vi "多参校准第二步.vi"(11 "校准模式":enum32{"单点校准", "多点校准"}(radio)) -> (1 "标样2浓度输出":dbl, 2 "标样1浓度输出":dbl, 3 "继续执行":bool)   [LabVIEW 2016, in "斯坦道仪器.lvlib"]
panel:
  in  "标样浓度 2":dbl
  in  "标样浓度":dbl
  in  "取消":bool
  in  "下一步":bool
  # "请输入标样一浓度："
  # "请输入标样二浓度："
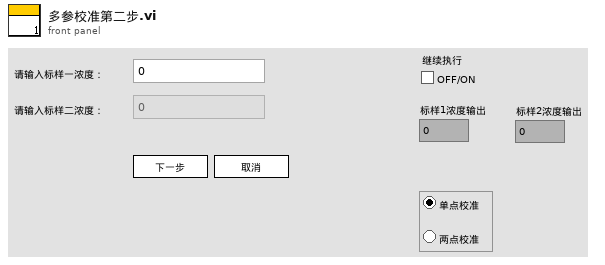
[diagram p1: front panel]
types:
  T1 = enum8{"Enabled", "Disabled", "Disabled and Grayed Out"}
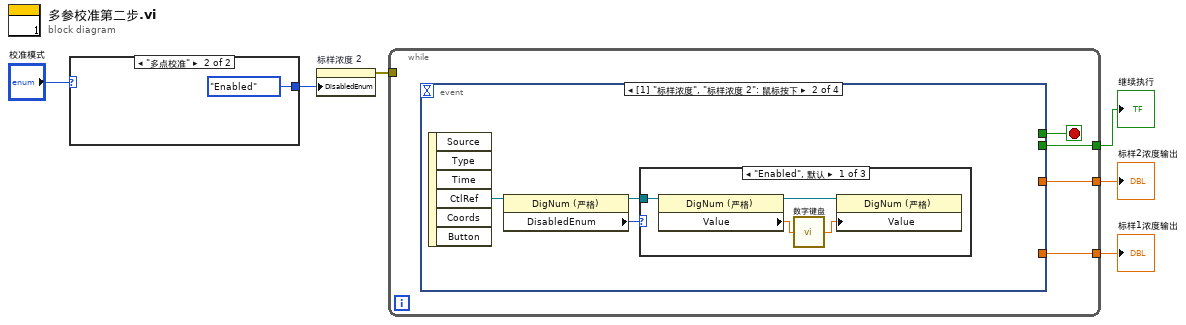
[diagram p0: block diagram]
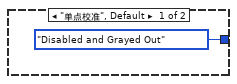
[diagram p2: hidden frame]
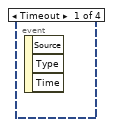
[diagram p3: hidden frame]
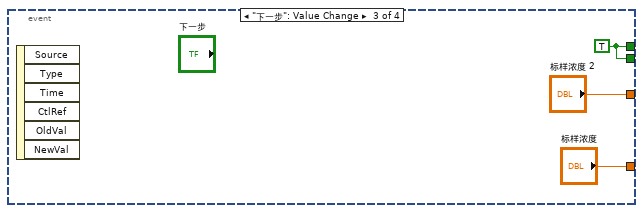
[diagram p6: hidden frame]
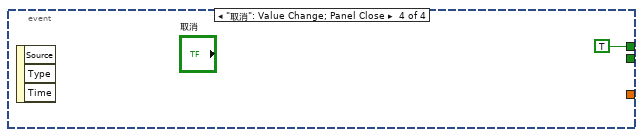
[diagram p7: hidden frame]
diagram:
  n1 = case shown="\"多点校准\"" "校准模式" {
    tunnel: [T1."Disabled and Grayed Out" ("禁用") T1."Enabled" ("禁用")] -> w1
    frame "单点校准", Default {
    }
    frame "多点校准" {
    }
  }
  n2 = property on="标样浓度 2" class="DigNum (严格)"("DisabledEnum"=w1) -> (error out=w2:errorcluster)  [unwired: 2 in, 1 out]
  n3 = while {
    tunnel: [w12] -> w6
    tunnel: [w10] -> w5
    tunnel: [w9] -> w4
    tunnel: w2 -> [_]
    stop <- w11 stop-if-true
    n4 = event shown="[1] \"标样浓度\", \"标样浓度 2\": 鼠标按下" {
      selector: _ -> [_ _ _ _]
      dyn-events: _ -> [_ _ _ _]
      timeout: _ -> [_ _ _ _]
      tunnel: [_ _ w22 _] -> w12
      tunnel: [_ _ w22 TRUE ("继续执行")] -> w11
      tunnel: [_ _ "标样浓度" _] -> w10
      tunnel: [_ _ "标样浓度 2" _] -> w9
      event Timeout {
        n5 = event-data() -> ()  [unwired: 1 in, 3 out]
      }
      event "标样浓度", "标样浓度 2": Mouse Down {
        n6 = event-data() -> ("CtlRef"=w15:refnum<vi>)  [unwired: 1 in, 5 out]
        n7 = property class="DigNum (严格)"(reference=w15) -> (reference out=w14:refnum<vi>, "DisabledEnum"=w13:T1)  [unwired: 1 in, 1 out]
        n8 = case shown="\"Enabled\", 默认" w13 {
          tunnel: w14 -> [w18 _ _]
          frame "Enabled", Default {
            n9 = property class="DigNum (严格)"(reference=w18) -> (reference out=w19:refnum<vi>, "Value"=w17:dbl)  [unwired: 1 in, 1 out]
            n10 = call "数字键盘.vi"("OldNumber"=w17) -> ("NewNumber"=w16:sgl)
            n11 = property class="DigNum (严格)"(reference=w19, "Value"=w16) -> ()  [unwired: 1 in, 2 out]
          }
          frame "Disabled" {
          }
          frame "Disabled and Grayed Out" {
          }
        }
      }
      event "下一步": Value Change {
        w22 = TRUE ("继续执行")
        n12 = event-data() -> ()  [unwired: 1 in, 6 out]
      }
      event "取消": Value Change; Panel Close {
        n13 = event-data() -> ()  [unwired: 1 in, 3 out]
      }
    }
  }
  "继续执行" <- w6
  "标样1浓度输出" <- w5
  "标样2浓度输出" <- w4
